vi "motorConfig.vi"(3 "Velocity":dbl=2.2, 4 "Acceleration":dbl=1.5, 5 "Device in":refnum<k24>) -> (2 "Device out":refnum<k24>)   [LabVIEW 2014]
doc: "André Romero - 2017\nandretec@ifsc.usp.br"
uses:
  C:/UserLabs/Andre/LabView2014-32bits/kinesisTec/Kinesis/Thorlabs.MotionControl.TCube.DCServoCLI.dll
  Kinesis/Thorlabs.MotionControl.TCube.DCServoCLI.dll
  C:/UserLabs/Andre/LabView2014-32bits/kinesisTec/Kinesis/Thorlabs.MotionControl.GenericMotorCLI.dll
  Kinesis/Thorlabs.MotionControl.GenericMotorCLI.dll
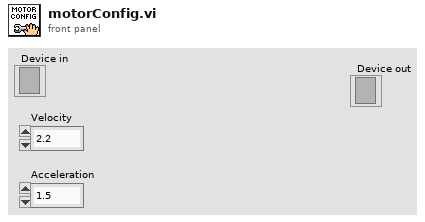
[diagram p1: front panel]
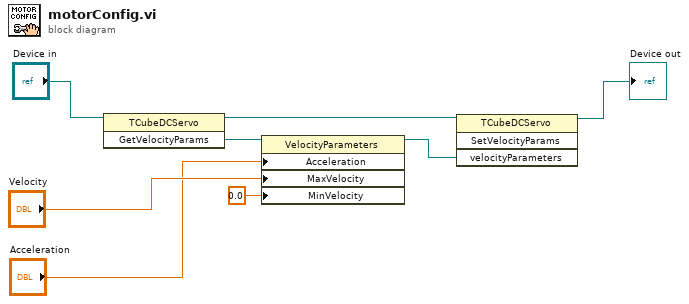
[diagram p0: block diagram]
diagram:
  n1 = invoke class="TCubeDCServo" method="GetVelocityParams"(reference="Device in") -> (reference out=w6:refnum<k24>, "GetVelocityParams"=w2:refnum<k24>)  [unwired: 2 in, 1 out]
  n2 = property class="VelocityParameters"(reference=w2, "Acceleration"="Acceleration", "MaxVelocity"="Velocity", "MinVelocity"=0.0) -> (reference out=w7:refnum<k24>)  [unwired: 1 in, 1 out]
  n3 = invoke class="TCubeDCServo" method="SetVelocityParams"(reference=w6, "velocityParameters"=w7) -> (reference out=→"Device out":refnum<k24>)  [unwired: 2 in, 3 out]
